vi "Function Generator--OLD.vi"(11 "Properties in":T1={"Schedule"=0, "Value"=0.0, "Start Value"=0.0, "End Value"=0.0, "Min Value"=0.0, "Max Value"=0.0, "Duty Cycle (%)"=0.0, "Speed Signal Type"=2, "Cycle Number"=0.0, "Phase (degrees)"=0.0} {"Schedule" items=["Constant", "Ramp", "Fn. Generator", "Formula"]; "Speed Signal Type" items=["Sine Wave", "Triangle Wave", "Square Wave", "Sawtooth Wave"]}) -> (2 "Properties out":T1={"Schedule"=0, "Value"=0.0, "Start Value"=0.0, "End Value"=0.0, "Min Value"=0.0, "Max Value"=0.0, "Duty Cycle (%)"=0.0, "Speed Signal Type"=2, "Cycle Number"=0.0, "Phase (degrees)"=0.0} {"Schedule" items=["Constant", "Ramp", "Fn. Generator", "Formula"]; "Speed Signal Type" items=["Sine Wave", "Triangle Wave", "Square Wave", "Sawtooth Wave"]}, 3 "Cancelled?":bool)   [LabVIEW 2019]
doc: "This VI is a dialog box that allows you to create a waveform for voltage/speed properties."
uses:
  <vilib>/measure/NI_MABase.lvlib
panel:
  in  "Samples (testing)":dbl=1000.0
  out "Signal":dbl[](graph)
  in  "Signal Type":u16(ring) items=["Sine Wave", "Triangle Wave", "Square Wave", "Sawtooth Wave"]
  in  "Phase (degrees)":dbl
  in  "Cycle Number":dbl
  in  "Square Wave\nDuty Cycle (%)":dbl
  in  "Max Value":dbl
  in  "Min Value":dbl
  in  "Cancel":bool
  in  "OK":bool
  # "Function Generator"
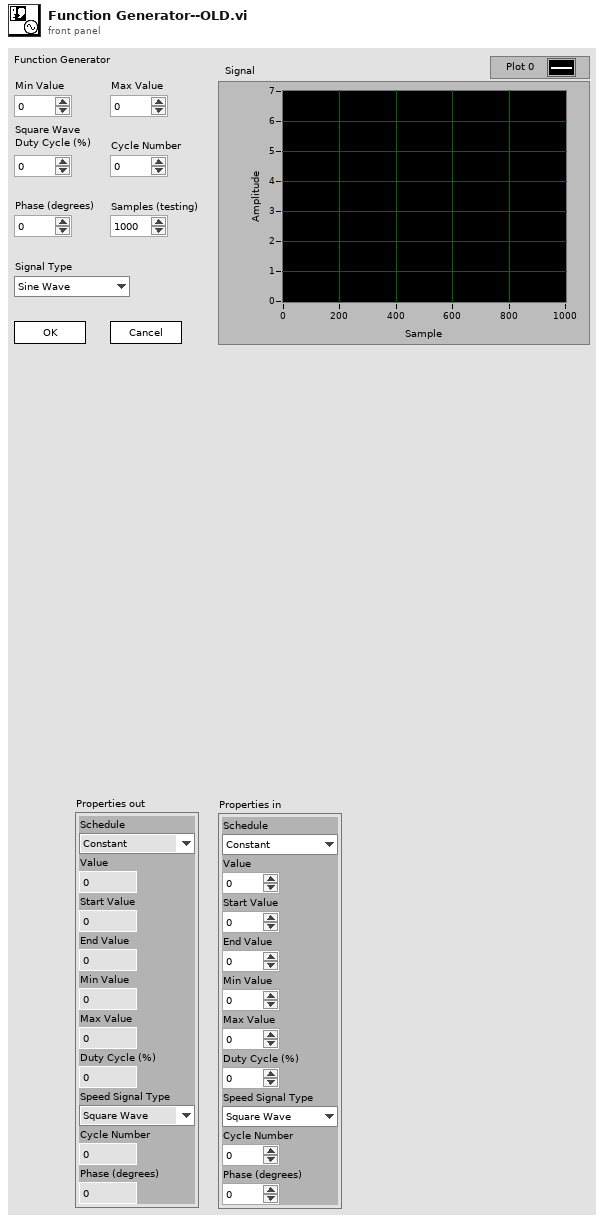
[diagram p1: front panel]
types:
  T1 = cluster{"Schedule":u16, "Value":dbl, "Start Value":dbl, "End Value":dbl, "Min Value":dbl, "Max Value":dbl, "Duty Cycle (%)":dbl, "Speed Signal Type":u16, "Cycle Number":dbl, "Phase (degrees)":dbl}
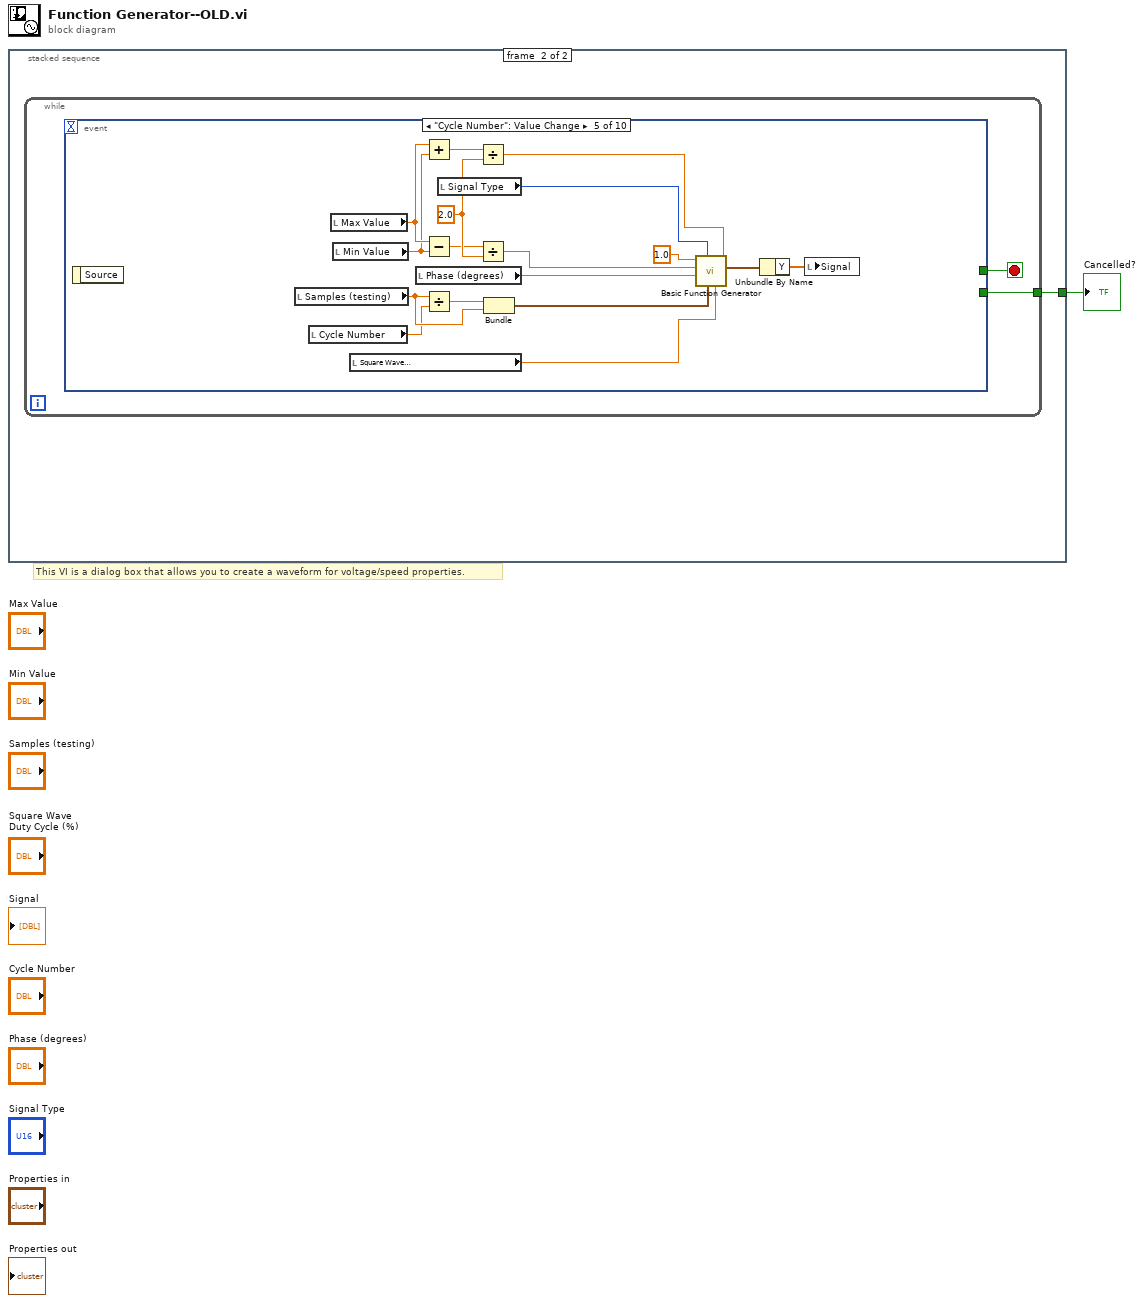
[diagram p0: block diagram]
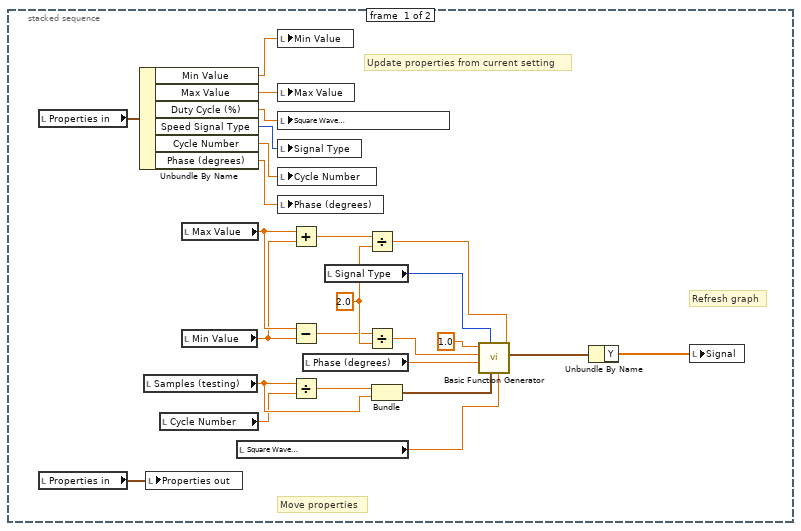
[diagram p2: hidden frame]
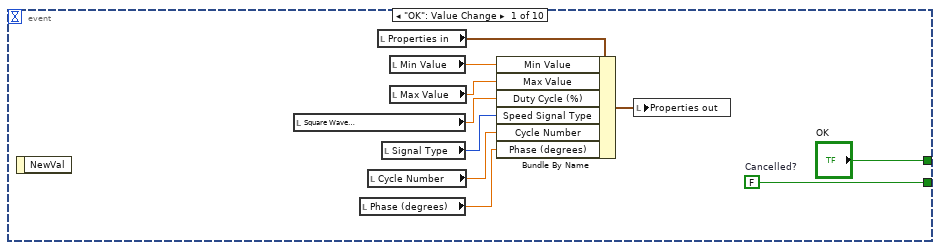
[diagram p3: hidden frame]
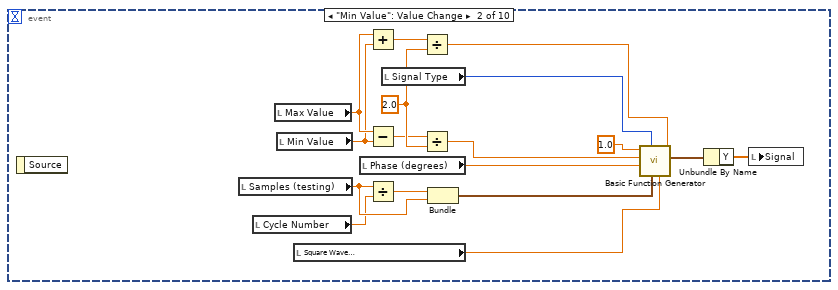
[diagram p4: hidden frame]
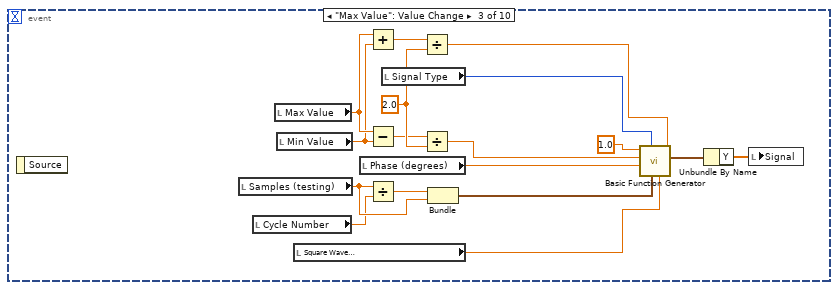
[diagram p5: hidden frame]
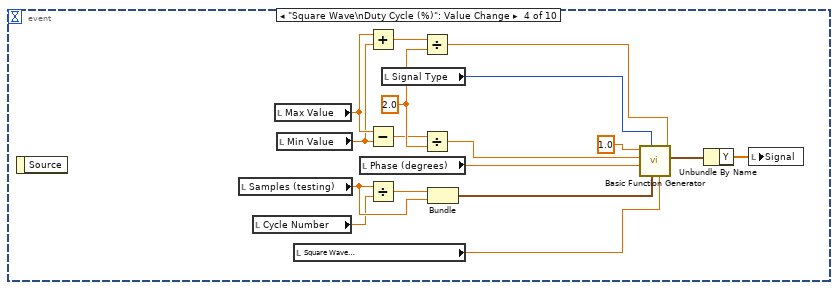
[diagram p6: hidden frame]
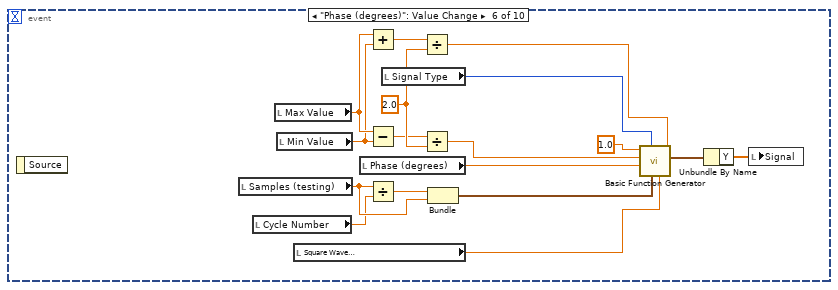
[diagram p7: hidden frame]
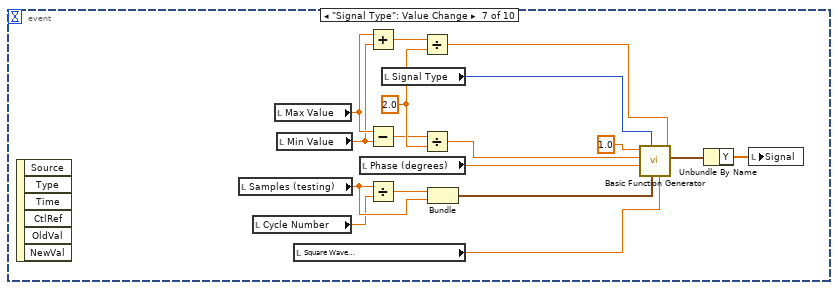
[diagram p8: hidden frame]
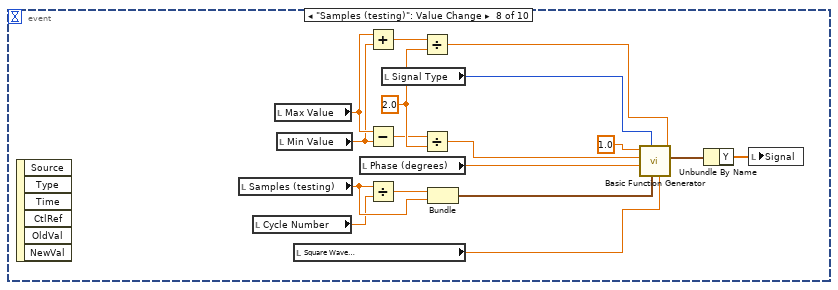
[diagram p9: hidden frame]
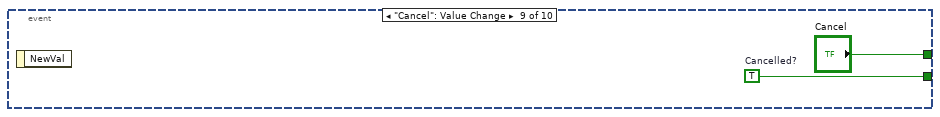
[diagram p10: hidden frame]
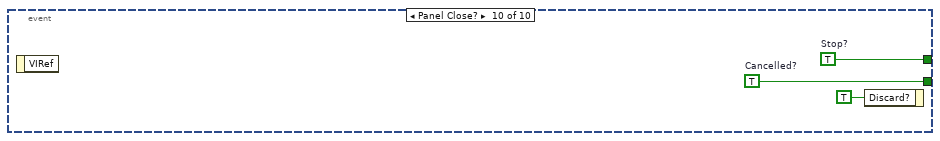
[diagram p11: hidden frame]
diagram:
  # "This VI is a dialog box that allows you to create a waveform for voltage/speed properties."
  n1 = stacked-sequence {
    tunnel: [_ w27] -> w1
    frame #0 {
      w15 = 2.0 ("y")
      # "Move properties"
      # "Update properties from current setting"
      # "Refresh graph"
      n2 = local read "Properties in"() -> (w26:T1)
      n3 = local read "Properties in"() -> (w2:T1)
      n4 = Unbundle By Name(w26) -> ("Min Value"=w25:dbl, "Max Value"=w24:dbl, "Duty Cycle (%)"=w23:dbl, "Speed Signal Type"=w22:u16, "Cycle Number"=w21:dbl, "Phase (degrees)"=w20:dbl)
      n5 = local read "Samples (testing)"() -> (w8:dbl)
      n6 = local write "Properties out"(w2) -> ()
      n7 = local read "Cycle Number"() -> (w7:dbl)
      n8 = local read "Max Value"() -> (w19:dbl)
      n9 = local read "Min Value"() -> (w6:dbl)
      n10 = local read "Square Wave\nDuty Cycle (%)"() -> (w4:dbl)
      n11 = local write "Min Value"(w25) -> ()
      n12 = local write "Max Value"(w24) -> ()
      n13 = local write "Square Wave\nDuty Cycle (%)"(w23) -> ()
      n14 = local write "Signal Type"(w22) -> ()
      n15 = local write "Cycle Number"(w21) -> ()
      n16 = local write "Phase (degrees)"(w20) -> ()
      n17 = Add(x=w19, y=w6) -> (x+y=w12:dbl)
      n18 = Subtract(x=w19, y=w6) -> (x-y=w14:dbl)
      n19 = Divide(x=w8, y=w7) -> (x/y=w18:dbl)
      n20 = local read "Phase (degrees)"() -> (w3:dbl)
      n21 = local read "Signal Type"() -> (w5:u16)
      n22 = Divide(x=w12, y=w15) -> (x/y=w13:dbl)
      n23 = Divide(x=w14, y=w15) -> (x/y=w16:dbl)
      n24 = Bundle(w18, "Samples (testing)"=w8) -> (w17:cluster{dbl, "Samples (testing)":dbl})  [unwired: 1 in]
      n25 = call <vilib>:"Basic Function Generator.vi"("offset"=w13, "square wave duty cycle (%)"=w4, "sampling info"=w17, "signal type"=w5, "phase"=w3, "amplitude"=w16, "frequency"=1.0) -> ("signal out"=w10:waveform(dbl))  [unwired: 2 in, 2 out]
      n26 = Unbundle By Name(w10) -> ("Y"=w9:dbl[])
      n27 = local write "Signal"(w9) -> ()
    }
    frame #1 {
      n28 = while {
        tunnel: [w28] -> w27
        stop <- w29 stop-if-true
        n29 = event shown="[4] \"Cycle Number\": Value Change" {
          selector: _ -> [_ _ _ _ _ _ _ _ _ _]
          dyn-events: _ -> [_ _ _ _ _ _ _ _ _ _]
          timeout: _ -> [_ _ _ _ _ _ _ _ _ _]
          tunnel: ["OK" _ _ _ _ _ _ _ "Cancel" w162] -> w29
          tunnel: [w39 _ _ _ _ _ _ _ w160 w161] -> w28
          event "OK": Value Change {
            w39 = FALSE  # Cancelled?
            n30 = event-data() -> ()  [unwired: 1 in, 1 out]
            n31 = local read "Square Wave\nDuty Cycle (%)"() -> (w35:dbl)
            n32 = local read "Phase (degrees)"() -> (w32:dbl)
            n33 = local read "Cycle Number"() -> (w33:dbl)
            n34 = local read "Properties in"() -> (w31:T1)
            n35 = local read "Signal Type"() -> (w34:u16)
            n36 = local read "Min Value"() -> (w37:dbl)
            n37 = local read "Max Value"() -> (w36:dbl)
            n38 = Bundle By Name(cluster=w31, "Min Value"=w37, "Max Value"=w36, "Duty Cycle (%)"=w35, "Speed Signal Type"=w34, "Cycle Number"=w33, "Phase (degrees)"=w32) -> (w30:T1)
            n39 = local write "Properties out"(w30) -> ()
          }
          event "Min Value": Value Change {
            w53 = 2.0 ("y")
            n40 = event-data() -> ()  [unwired: 1 in, 1 out]
            n41 = local read "Samples (testing)"() -> (w46:dbl)
            n42 = local read "Cycle Number"() -> (w45:dbl)
            n43 = local read "Max Value"() -> (w44:dbl)
            n44 = local read "Min Value"() -> (w43:dbl)
            n45 = local read "Square Wave\nDuty Cycle (%)"() -> (w41:dbl)
            n46 = local read "Phase (degrees)"() -> (w40:dbl)
            n47 = Add(x=w44, y=w43) -> (x+y=w50:dbl)
            n48 = Subtract(x=w44, y=w43) -> (x-y=w52:dbl)
            n49 = Divide(x=w46, y=w45) -> (x/y=w56:dbl)
            n50 = local read "Signal Type"() -> (w42:u16)
            n51 = Divide(x=w50, y=w53) -> (x/y=w51:dbl)
            n52 = Divide(x=w52, y=w53) -> (x/y=w54:dbl)
            n53 = Bundle(w56, "Samples (testing)"=w46) -> (w55:cluster{dbl, "Samples (testing)":dbl})  [unwired: 1 in]
            n54 = call <vilib>:"Basic Function Generator.vi"("offset"=w51, "square wave duty cycle (%)"=w41, "sampling info"=w55, "signal type"=w42, "phase"=w40, "amplitude"=w54, "frequency"=1.0) -> ("signal out"=w48:waveform(dbl))  [unwired: 2 in, 2 out]
            n55 = Unbundle By Name(w48) -> ("Y"=w47:dbl[])
            n56 = local write "Signal"(w47) -> ()
          }
          event "Max Value": Value Change {
            w70 = 2.0 ("y")
            n57 = event-data() -> ()  [unwired: 1 in, 1 out]
            n58 = local read "Samples (testing)"() -> (w63:dbl)
            n59 = local read "Cycle Number"() -> (w62:dbl)
            n60 = local read "Max Value"() -> (w61:dbl)
            n61 = local read "Min Value"() -> (w60:dbl)
            n62 = local read "Square Wave\nDuty Cycle (%)"() -> (w58:dbl)
            n63 = local read "Phase (degrees)"() -> (w57:dbl)
            n64 = Add(x=w61, y=w60) -> (x+y=w67:dbl)
            n65 = Subtract(x=w61, y=w60) -> (x-y=w69:dbl)
            n66 = Divide(x=w63, y=w62) -> (x/y=w73:dbl)
            n67 = local read "Signal Type"() -> (w59:u16)
            n68 = Divide(x=w67, y=w70) -> (x/y=w68:dbl)
            n69 = Divide(x=w69, y=w70) -> (x/y=w71:dbl)
            n70 = Bundle(w73, "Samples (testing)"=w63) -> (w72:cluster{dbl, "Samples (testing)":dbl})  [unwired: 1 in]
            n71 = call <vilib>:"Basic Function Generator.vi"("offset"=w68, "square wave duty cycle (%)"=w58, "sampling info"=w72, "signal type"=w59, "phase"=w57, "amplitude"=w71, "frequency"=1.0) -> ("signal out"=w65:waveform(dbl))  [unwired: 2 in, 2 out]
            n72 = Unbundle By Name(w65) -> ("Y"=w64:dbl[])
            n73 = local write "Signal"(w64) -> ()
          }
          event "Square Wave\nDuty Cycle (%)": Value Change {
            w87 = 2.0 ("y")
            n74 = event-data() -> ()  [unwired: 1 in, 1 out]
            n75 = local read "Samples (testing)"() -> (w80:dbl)
            n76 = local read "Cycle Number"() -> (w79:dbl)
            n77 = local read "Max Value"() -> (w78:dbl)
            n78 = local read "Min Value"() -> (w77:dbl)
            n79 = local read "Square Wave\nDuty Cycle (%)"() -> (w75:dbl)
            n80 = local read "Phase (degrees)"() -> (w74:dbl)
            n81 = Add(x=w78, y=w77) -> (x+y=w84:dbl)
            n82 = Subtract(x=w78, y=w77) -> (x-y=w86:dbl)
            n83 = Divide(x=w80, y=w79) -> (x/y=w90:dbl)
            n84 = local read "Signal Type"() -> (w76:u16)
            n85 = Divide(x=w84, y=w87) -> (x/y=w85:dbl)
            n86 = Divide(x=w86, y=w87) -> (x/y=w88:dbl)
            n87 = Bundle(w90, "Samples (testing)"=w80) -> (w89:cluster{dbl, "Samples (testing)":dbl})  [unwired: 1 in]
            n88 = call <vilib>:"Basic Function Generator.vi"("offset"=w85, "square wave duty cycle (%)"=w75, "sampling info"=w89, "signal type"=w76, "phase"=w74, "amplitude"=w88, "frequency"=1.0) -> ("signal out"=w82:waveform(dbl))  [unwired: 2 in, 2 out]
            n89 = Unbundle By Name(w82) -> ("Y"=w81:dbl[])
            n90 = local write "Signal"(w81) -> ()
          }
          event "Cycle Number": Value Change {
            w104 = 2.0 ("y")
            n91 = event-data() -> ()  [unwired: 1 in, 1 out]
            n92 = local read "Samples (testing)"() -> (w97:dbl)
            n93 = local read "Cycle Number"() -> (w96:dbl)
            n94 = local read "Max Value"() -> (w95:dbl)
            n95 = local read "Min Value"() -> (w94:dbl)
            n96 = local read "Square Wave\nDuty Cycle (%)"() -> (w92:dbl)
            n97 = local read "Phase (degrees)"() -> (w91:dbl)
            n98 = Add(x=w95, y=w94) -> (x+y=w101:dbl)
            n99 = Subtract(x=w95, y=w94) -> (x-y=w103:dbl)
            n100 = Divide(x=w97, y=w96) -> (x/y=w107:dbl)
            n101 = local read "Signal Type"() -> (w93:u16)
            n102 = Divide(x=w101, y=w104) -> (x/y=w102:dbl)
            n103 = Divide(x=w103, y=w104) -> (x/y=w105:dbl)
            n104 = Bundle(w107, "Samples (testing)"=w97) -> (w106:cluster{dbl, "Samples (testing)":dbl})  [unwired: 1 in]
            n105 = call <vilib>:"Basic Function Generator.vi"("offset"=w102, "square wave duty cycle (%)"=w92, "sampling info"=w106, "signal type"=w93, "phase"=w91, "amplitude"=w105, "frequency"=1.0) -> ("signal out"=w99:waveform(dbl))  [unwired: 2 in, 2 out]
            n106 = Unbundle By Name(w99) -> ("Y"=w98:dbl[])
            n107 = local write "Signal"(w98) -> ()
          }
          event "Phase (degrees)": Value Change {
            w121 = 2.0 ("y")
            n108 = event-data() -> ()  [unwired: 1 in, 1 out]
            n109 = local read "Samples (testing)"() -> (w114:dbl)
            n110 = local read "Cycle Number"() -> (w113:dbl)
            n111 = local read "Max Value"() -> (w112:dbl)
            n112 = local read "Min Value"() -> (w111:dbl)
            n113 = local read "Square Wave\nDuty Cycle (%)"() -> (w109:dbl)
            n114 = local read "Phase (degrees)"() -> (w108:dbl)
            n115 = Add(x=w112, y=w111) -> (x+y=w118:dbl)
            n116 = Subtract(x=w112, y=w111) -> (x-y=w120:dbl)
            n117 = Divide(x=w114, y=w113) -> (x/y=w124:dbl)
            n118 = local read "Signal Type"() -> (w110:u16)
            n119 = Divide(x=w118, y=w121) -> (x/y=w119:dbl)
            n120 = Divide(x=w120, y=w121) -> (x/y=w122:dbl)
            n121 = Bundle(w124, "Samples (testing)"=w114) -> (w123:cluster{dbl, "Samples (testing)":dbl})  [unwired: 1 in]
            n122 = call <vilib>:"Basic Function Generator.vi"("offset"=w119, "square wave duty cycle (%)"=w109, "sampling info"=w123, "signal type"=w110, "phase"=w108, "amplitude"=w122, "frequency"=1.0) -> ("signal out"=w116:waveform(dbl))  [unwired: 2 in, 2 out]
            n123 = Unbundle By Name(w116) -> ("Y"=w115:dbl[])
            n124 = local write "Signal"(w115) -> ()
          }
          event "Signal Type": Value Change {
            w138 = 2.0 ("y")
            n125 = event-data() -> ()  [unwired: 1 in, 6 out]
            n126 = local read "Samples (testing)"() -> (w131:dbl)
            n127 = local read "Cycle Number"() -> (w130:dbl)
            n128 = local read "Max Value"() -> (w129:dbl)
            n129 = local read "Min Value"() -> (w128:dbl)
            n130 = local read "Square Wave\nDuty Cycle (%)"() -> (w126:dbl)
            n131 = local read "Phase (degrees)"() -> (w125:dbl)
            n132 = Add(x=w129, y=w128) -> (x+y=w135:dbl)
            n133 = Subtract(x=w129, y=w128) -> (x-y=w137:dbl)
            n134 = Divide(x=w131, y=w130) -> (x/y=w141:dbl)
            n135 = local read "Signal Type"() -> (w127:u16)
            n136 = Divide(x=w135, y=w138) -> (x/y=w136:dbl)
            n137 = Divide(x=w137, y=w138) -> (x/y=w139:dbl)
            n138 = Bundle(w141, "Samples (testing)"=w131) -> (w140:cluster{dbl, "Samples (testing)":dbl})  [unwired: 1 in]
            n139 = call <vilib>:"Basic Function Generator.vi"("offset"=w136, "square wave duty cycle (%)"=w126, "sampling info"=w140, "signal type"=w127, "phase"=w125, "amplitude"=w139, "frequency"=1.0) -> ("signal out"=w133:waveform(dbl))  [unwired: 2 in, 2 out]
            n140 = Unbundle By Name(w133) -> ("Y"=w132:dbl[])
            n141 = local write "Signal"(w132) -> ()
          }
          event "Samples (testing)": Value Change {
            w155 = 2.0 ("y")
            n142 = event-data() -> ()  [unwired: 1 in, 6 out]
            n143 = local read "Samples (testing)"() -> (w148:dbl)
            n144 = local read "Cycle Number"() -> (w147:dbl)
            n145 = local read "Max Value"() -> (w146:dbl)
            n146 = local read "Min Value"() -> (w145:dbl)
            n147 = local read "Square Wave\nDuty Cycle (%)"() -> (w143:dbl)
            n148 = local read "Phase (degrees)"() -> (w142:dbl)
            n149 = Add(x=w146, y=w145) -> (x+y=w152:dbl)
            n150 = Subtract(x=w146, y=w145) -> (x-y=w154:dbl)
            n151 = Divide(x=w148, y=w147) -> (x/y=w158:dbl)
            n152 = local read "Signal Type"() -> (w144:u16)
            n153 = Divide(x=w152, y=w155) -> (x/y=w153:dbl)
            n154 = Divide(x=w154, y=w155) -> (x/y=w156:dbl)
            n155 = Bundle(w158, "Samples (testing)"=w148) -> (w157:cluster{dbl, "Samples (testing)":dbl})  [unwired: 1 in]
            n156 = call <vilib>:"Basic Function Generator.vi"("offset"=w153, "square wave duty cycle (%)"=w143, "sampling info"=w157, "signal type"=w144, "phase"=w142, "amplitude"=w156, "frequency"=1.0) -> ("signal out"=w150:waveform(dbl))  [unwired: 2 in, 2 out]
            n157 = Unbundle By Name(w150) -> ("Y"=w149:dbl[])
            n158 = local write "Signal"(w149) -> ()
          }
          event "Cancel": Value Change {
            w160 = TRUE  # Cancelled?
            n159 = event-data() -> ()  [unwired: 1 in, 1 out]
          }
          event Panel Close? {
            w161 = TRUE  # Cancelled?
            w162 = TRUE  # Stop?
            n160 = event-data() -> ()  [unwired: 1 in, 1 out]
            n161 = event-data("Discard?"=TRUE) -> ()  [unwired: 1 in, 1 out]
          }
        }
      }
    }
  }
  "Cancelled?" <- w1
